vi "Main Engine Stream Process.vi"(8 "error in (no error)":errorcluster, 10 "Refs":T1 {"Termination" items=["Off", "On"]}, 11 "Process in":refnum<class "Process.lvclass">) -> (0 "error out":errorcluster)   [LabVIEW 2019, in "CAN Stream Support Engine.lvlib"]
uses:
  CAN Stream Support Engine.lvlib
  <vilib>/NI/NIVS Inline Async API/_VS Inline Async API/Process/Process.lvclass
  Types/Engine Stream Refs.ctl
  Addon Shared/Types/Direction Filter.ctl
  Addon Shared/Types/Type Filter.ctl
  Addon Shared/Types/Filter Parameters.ctl
  Types/Engine Stream State.ctl
  Addon Shared/Types/Stream Type.ctl
  <vilib>/xnet/xnet.llb/XNET CAN Comm.ctl
  <vilib>/xnet/xnet.llb/XNET CAN Comm State.ctl
  <vilib>/xnet/xnet.llb/XNET CAN Last Err.ctl
  <vilib>/xnet/xnet.llb/XNET Frame CAN.ctl
  <vilib>/xnet/xnet.llb/XNET Frame Type CAN.ctl
  <vilib>/NI/NIVS Inline Async API/_VS Inline Async API/Process/Process.lvclass/Process.ctl
  <vilib>/NI/NIVS Inline Async API/_VS Inline Async API/Error Handling Process/SubVIs/Error.ConvertArray.vi
  <vilib>/xnet/xnet.llb/XNET Create Session (Frame Input Stream).vi
  <vilib>/Utility/SystemLogging/Write to System Log.vi
  <vilib>/xnet/xnet.llb/XNET Read (Frame CAN).vi
  <vilib>/xnet/xnet.llb/XNET Read (State CAN Comm).vi
  <resource>/objmgr/xnet.rc
  Addon Shared/CAN Stream Support Shared.lvlib
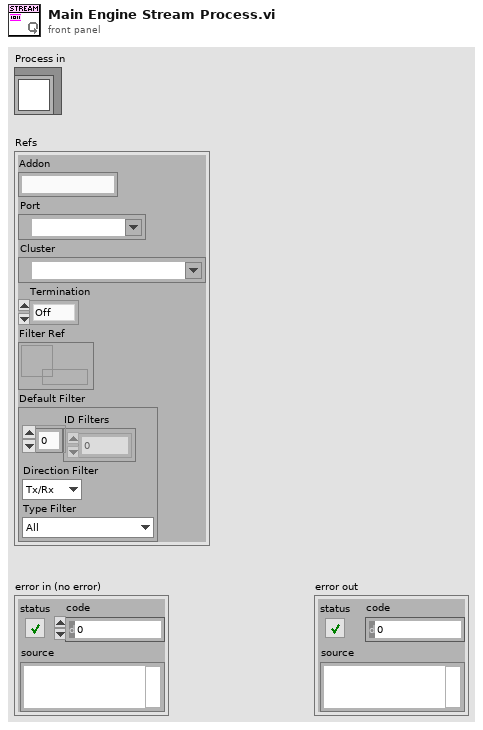
[diagram p1: front panel]
types:
  T1 = typedef "CAN Stream Support Engine.lvlib/Engine Stream Refs.ctl" = cluster{"Addon":string, "Port":refnum<k21>, "Cluster":refnum<k21>, "Termination":u32, "Filter Ref":refnum<data-value>, "Default Filter":T2}
  T2 = typedef "CAN Stream Support Shared.lvlib/Filter Parameters.ctl" = cluster{"ID Filters":u32[], "Direction Filter":T3, "Type Filter":T4}
  T3 = typedef "CAN Stream Support Shared.lvlib/Direction Filter.ctl" = enum16{"Tx/Rx", "Rx", "Tx"}
  T4 = typedef "CAN Stream Support Shared.lvlib/Type Filter.ctl" = enum16{"All", "CAN Data", "CAN Remote", "CAN Bus Error", "CAN 2.0 Data", "CAN FD Data", "CAN FD+BRS Data", "J1939 Data", "Delay", "Log Trigger", "Start Trigger"}
  T5 = typedef "CAN Stream Support Engine.lvlib/Engine Stream State.ctl" = enum8{"Check for Connection", "Open XNET Session", "Publish", "Cleanup", "Exit"}
  T6 = typedef "CAN Stream Support Shared.lvlib/Stream Type.ctl" = cluster{"State":T7, "Frames":T10[]}
  T7 = typedef "XNET CAN Comm.ctl" = cluster{"fault code":i32, "fault?":bool, "communication state":T8, "last error":T9, "receive error counter":u8, "transmit error counter":u8, "transceiver error?":bool, "sleep?":bool}
  T8 = typedef "XNET CAN Comm State.ctl" = u8
  T9 = typedef "XNET CAN Last Err.ctl" = u8
  T10 = typedef "XNET Frame CAN.ctl" = cluster{"timestamp":timestamp, "payload":u8[], "identifier":u32, "type":T11, "extended?":bool, "echo?":bool}
  T11 = typedef "XNET Frame Type CAN.ctl" = u8
  T12 = cluster{"ID Filters":u32[], "Direction Filter":T3, "Type Filter":T4}
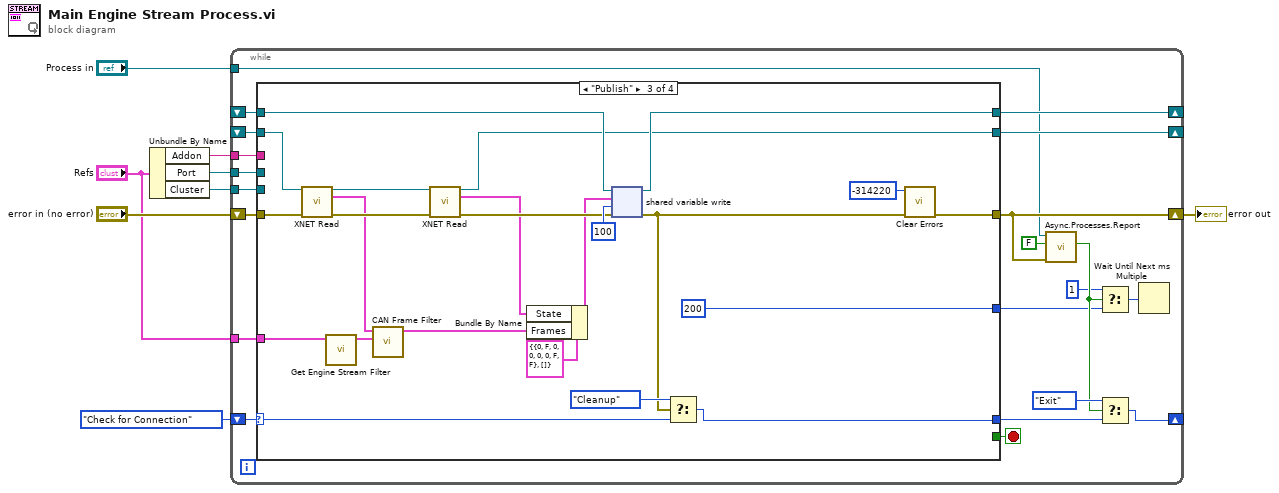
[diagram p0: block diagram]
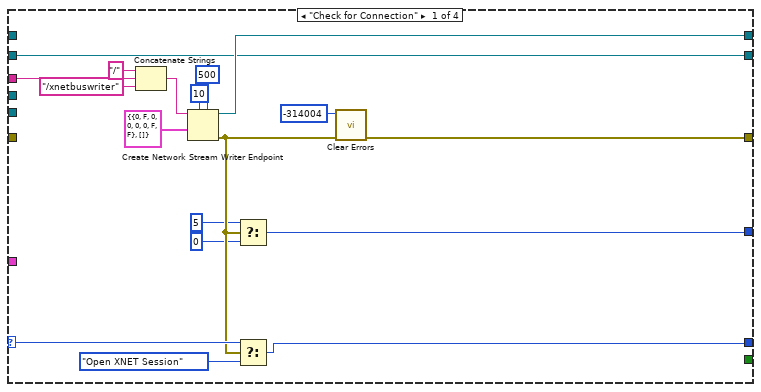
[diagram p2: hidden frame]
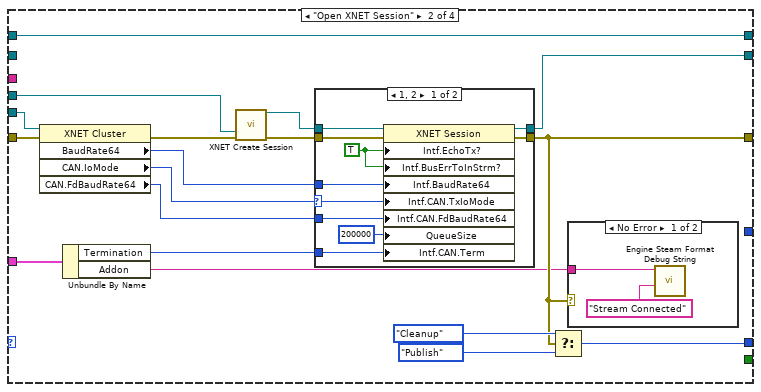
[diagram p3: hidden frame]
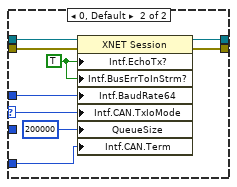
[diagram p4: hidden frame]
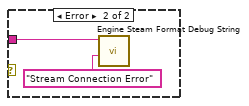
[diagram p5: hidden frame]
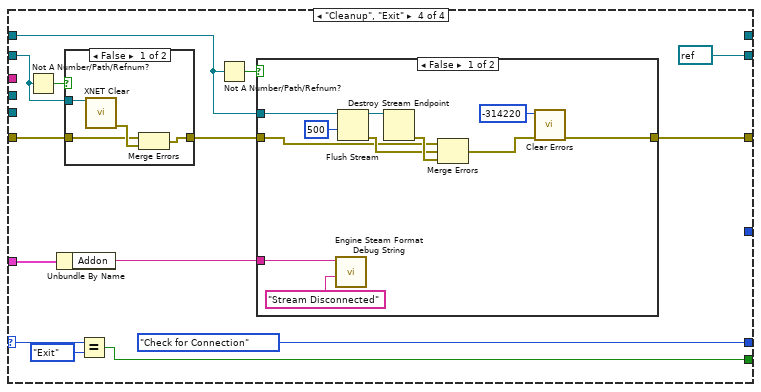
[diagram p6: hidden frame]
diagram:
  n1 = Unbundle By Name("Refs") -> ("Addon"=w3:string, "Port"=w1:refnum<k21>, "Cluster"=w2:refnum<k21>)
  n2 = while {
    shift-right: [w14] -> _
    shift-left: Engine_Stream_State."Check for Connection" -> [w29]
    shift-right: [w28] -> _
    shift-left: _ -> [w27]
    shift-right: [w21] -> w6
    shift-left: "error in (no error)" -> [w26]
    tunnel: w1 -> [w15]
    shift-right: [w24] -> _
    shift-left: _ -> [w23]
    tunnel: w2 -> [w22]
    tunnel: "Process in" -> [w18]
    tunnel: "Refs" -> [w17]
    tunnel: w3 -> [w16]
    stop <- w25 stop-if-true
    n3 = case shown="\"Publish\"" w29 {
      selector: w29 -> [w45 _ w108 w124]
      tunnel: [w43 w62 w107 Engine_Stream_State."Check for Connection"] -> w19
      tunnel: [w42 w63 w109 _] -> w28
      tunnel: w27 -> [_ w63 w110 w121]
      tunnel: [w40 w58 w92 w114] -> w21
      tunnel: w26 -> [_ w57 w103 w116]
      tunnel: [_ _ _ w122] -> w25
      tunnel: [w41 w60 w98 refnum<k21> refnum ("session out")] -> w24
      tunnel: w23 -> [w41 _ w105 w118]
      tunnel: [w34 _ u32 200 ("millisecond multiple") _] -> w12
      tunnel: w22 -> [_ w56 _ _]
      tunnel: w17 -> [_ w51 w102 w113]
      tunnel: w16 -> [w31 _ _ _]
      tunnel: w15 -> [_ w48 _ _]
      frame "Check for Connection" {
        n4 = Concatenate Strings("/" ("string"), w31, "/xnetbuswriter" ("reader url")) -> (w30:string)
        n5 = Create Network Stream Writer Endpoint(5:500 ("timeout in ms (-1)"), 7:10 ("writer buffer size"), 9:T6 {"State"={"fault code"=0, "fault?"=FALSE, "communication state"=0, "last error"=0, "receive error counter"=0, "transmit error counter"=0, "transceiver error?"=FALSE, "sleep?"=FALSE}, "Frames"=[]} ("Stream"), 11:w30) -> (0:w37:errorcluster, 3:w42:refnum<k21>)  [unwired: 3 in]
        n6 = Select(t=u32 5 ("millisecond multiple"), s=w37, f=u32 0) -> (s? t:f=w34:u32)
        n7 = Select(t=w45, s=w37, f=Engine_Stream_State."Open XNET Session") -> (s? t:f=w43:T5)
        n8 = call <vilib>:"Clear Errors.vi"("error in (no error)"=w37, "specific error code to clear (0: all)"=-314004) -> ("error out"=w40:errorcluster)  [unwired: 4 in, 1 out]
      }
      frame "Open XNET Session" {
        n9 = property class="XNET Cluster"(reference=w56, error in=w57) -> (error out=w55:errorcluster, "BaudRate64"=w54:u64, "CAN.IoMode"=w53:u32, "CAN.FdBaudRate64"=w52:u64)  [unwired: 1 out]
        n10 = Unbundle By Name(w51) -> ("Termination"=w49:u32, "Addon"=w50:string)
        n11 = call-poly <vilib>:"XNET Create Session.vi"("interface"=w48, "error in (no error)"=w55) -> ("session out"=w61:refnum<k21>, "error out"=w59:errorcluster)  [unwired: 1 in, 11 out]
        n12 = case shown="1, 2" w53 {
          selector: w53 -> [w70 w79]
          tunnel: w61 -> [w75 w84]
          tunnel: [w74 w83] -> w60
          tunnel: w59 -> [w73 w82]
          tunnel: [w72 w81] -> w58
          tunnel: w54 -> [w71 w80]
          tunnel: w52 -> [w69 _]
          tunnel: w49 -> [w68 w78]
          frame 1, 2 {
            w66 = TRUE ("Interface:Echo Transmit?")
            n13 = property class="XNET Session"(reference=w75, error in=w73, "Intf.EchoTx?"=w66, "Intf.BusErrToInStrm?"=w66, "Intf.BaudRate64"=w71, "Intf.CAN.TxIoMode"=w70, "Intf.CAN.FdBaudRate64"=w69, "QueueSize"=u32 200000 ("Queue Size"), "Intf.CAN.Term"=w68) -> (reference out=w74:refnum<k21>, error out=w72:errorcluster)
          }
          frame 0, Default {
            w76 = TRUE ("Interface:Echo Transmit?")
            n14 = property class="XNET Session"(reference=w84, error in=w82, "Intf.EchoTx?"=w76, "Intf.BusErrToInStrm?"=w76, "Intf.BaudRate64"=w80, "Intf.CAN.TxIoMode"=w79, "QueueSize"=u32 200000 ("Queue Size"), "Intf.CAN.Term"=w78) -> (reference out=w83:refnum<k21>, error out=w81:errorcluster)
          }
        }
        n15 = Select(t=Engine_Stream_State."Cleanup", s=w58, f=Engine_Stream_State."Publish") -> (s? t:f=w62:T5)
        n16 = case shown="No Error" w58 {
          tunnel: w50 -> [w85 w87]
          frame No Error {
            n17 = call "Engine Steam Format Debug String.vi"("State"="Stream Connected", "Name"=w85) -> ()  [unwired: 9 in, 1 out]
          }
          frame Error {
            n18 = call "Engine Steam Format Debug String.vi"("State"="Stream Connection Error", "Name"=w87) -> ()  [unwired: 9 in, 1 out]
          }
        }
      }
      frame "Publish" {
        n19 = call-poly <vilib>:"XNET Read.vi"("session in"=w105, "error in (no error)"=w103) -> ("session out"=w99:refnum<k21>, "data"=w91:T10[], "error out"=w101:errorcluster)  [unwired: 11 out]
        n20 = call "Get Engine Stream Filter.vi"("Refs"=w102) -> ("Filter"=w89:T12)  [unwired: 9 in, 1 out]
        n21 = call "CAN Frame Filter.vi"("Filter"=w89, "frames in"=w91) -> ("frames out"=w90:T10[])  [unwired: 9 in]
        n22 = call-poly <vilib>:"XNET Read.vi"("session in"=w99, "error in (no error)"=w101) -> ("session out"=w98:refnum<k21>, "CAN comm"=w97:T7, "error out"=w100:errorcluster)  [unwired: 11 out]
        n23 = Bundle By Name(cluster=T6 {"State"={"fault code"=0, "fault?"=FALSE, "communication state"=0, "last error"=0, "receive error counter"=0, "transmit error counter"=0, "transceiver error?"=FALSE, "sleep?"=FALSE}, "Frames"=[]} ("Stream"), "State"=w97, "Frames"=w90) -> (w96:T6)
        n24 = shared-variable-write(w110, w100, w96, 100 ("timeout ms")) -> (w109:refnum<k21>, w93:errorcluster)  [unwired: 1 out]
        n25 = Select(t=Engine_Stream_State."Cleanup", s=w93, f=w108) -> (s? t:f=w107:T5)
        n26 = call <vilib>:"Clear Errors.vi"("error in (no error)"=w93, "specific error code to clear (0: all)"=-314220) -> ("error out"=w92:errorcluster)  [unwired: 4 in, 1 out]
      }
      frame "Cleanup", "Exit" {
        n27 = Not A Number/Path/Refnum?(number/path/refnum=w118) -> (NaN/Path/Refnum?=w117:bool)
        n28 = Unbundle By Name(w113) -> ("Addon"=w112:string)
        n29 = case shown="False" w117 {
          tunnel: w116 -> [w126 w130]
          tunnel: [w127 w130] -> w115
          tunnel: w118 -> [w129 _]
          frame False {
            n30 = call <vilib>:"XNET Clear.vi"("session in"=w129) -> ("error out"=w128:errorcluster)  [unwired: 14 in]
            n31 = Merge Errors(w126, w128) -> (w127:errorcluster)
          }
          frame True {
          }
        }
        n32 = Equal?(x=w124, y=Engine_Stream_State."Exit") -> (x = y?=w122:bool)
        n33 = Not A Number/Path/Refnum?(number/path/refnum=w121) -> (NaN/Path/Refnum?=w120:bool)
        n34 = case shown="False" w120 {
          tunnel: w115 -> [w134 w142]
          tunnel: [w131 w142] -> w114
          tunnel: w121 -> [w140 _]
          tunnel: w112 -> [w138 _]
          frame False {
            n35 = call "Engine Steam Format Debug String.vi"("State"="Stream Disconnected", "Name"=w138) -> ()  [unwired: 9 in, 1 out]
            n36 = Flush Stream(9:500 ("timeout in ms (-1)"), 11:w140) -> (0:w135:errorcluster, 3:w141:refnum<k21>)  [unwired: 2 in, 1 out]
            n37 = Destroy Stream Endpoint(11:w141) -> (0:w137:errorcluster)  [unwired: 1 in]
            n38 = Merge Errors(w134, w135, w137) -> (w132:errorcluster)
            n39 = call <vilib>:"Clear Errors.vi"("error in (no error)"=w132, "specific error code to clear (0: all)"=-314220) -> ("error out"=w131:errorcluster)  [unwired: 4 in, 1 out]
          }
          frame True {
          }
        }
      }
    }
    n40 = call <vilib>:"Async.Processes.Report.vi"("Error"=w21, "Stop Async on Error?"=FALSE, "Process in"=w18) -> ("Stop"=w13:bool)  [unwired: 7 in, 1 out]
    n41 = Select(t=u32 1, s=w13, f=w12) -> (s? t:f=w11:u32)
    n42 = Select(t=Engine_Stream_State."Exit" ("y"), s=w13, f=w19) -> (s? t:f=w14:T5)
    n43 = Wait Until Next ms Multiple(millisecond multiple=w11) -> ()  [unwired: 1 out]
  }
  "error out" <- w6
